vi "MeasureMaxPStab_v2.vi"(7 "Scan Settings JV":T1={"Light intensity (Suns)"=1.0, "Pre-bias time (s)"=0.0, "Maximum voltage (V)"=0.0, "Minimum voltage (V)"=-1.4, "Range Options"=4, "1st scan FB to SC?"=TRUE, "Step Size (V)"=0.01, "Source Delay (s)"=0.01, "Inverted device"=FALSE, "Measure stabilized power output"=TRUE, "Stabilzation time (s)"=40.0, "Use Vmp from JV scan"=TRUE, "Stabization voltage (V)"=0.8, "Only stabilize best pixels"=TRUE, "Number of pixels to stabilize \nper substrate"=0, "Stabilization time step (s)"=1.0, "Use max power tracking"=FALSE, "Pre-bias voltage (V)"=-1.4, "No. of data point averages"=1.0, "No. of J-V averages"=1.0, "Integration time (ms)"=200.0} {"Number of pixels to stabilize \nper substrate" items=["1", "2", "3", "4", "5", "6", "7", "8"]; "Range Options" items=["Auto Range", "100 uA", "1 mA", "10 mA", "100 mA", "1A"]}, 9 "Voltage List":dbl[](array[numeric])) -> (0 "error out":errorcluster, 1 "Data Array":dbl[][](array[numeric]), 3 "VISA resource name out":refnum<visa-resource-name>)   [LabVIEW 2011]
uses:
  Typedefs/Scan settings.ctl
  <instrlib>/Keithley 24XX/Public/Data/Read (Multiple Points).vi
  <instrlib>/Keithley 24XX/Keithley 24XX.lvlib
panel:
  in  "Manual Range (1.0)":dbl=1.0
  in  "Source Mode  (0: Voltage)":u16(ring) items=["Voltage", "Current"]
  in  "VISA resource name":refnum<visa-resource-name>="GPIB0::24::INSTR"
  in  "Number of Points":u32=5
  in  "Compliance  Level":dbl=0.1
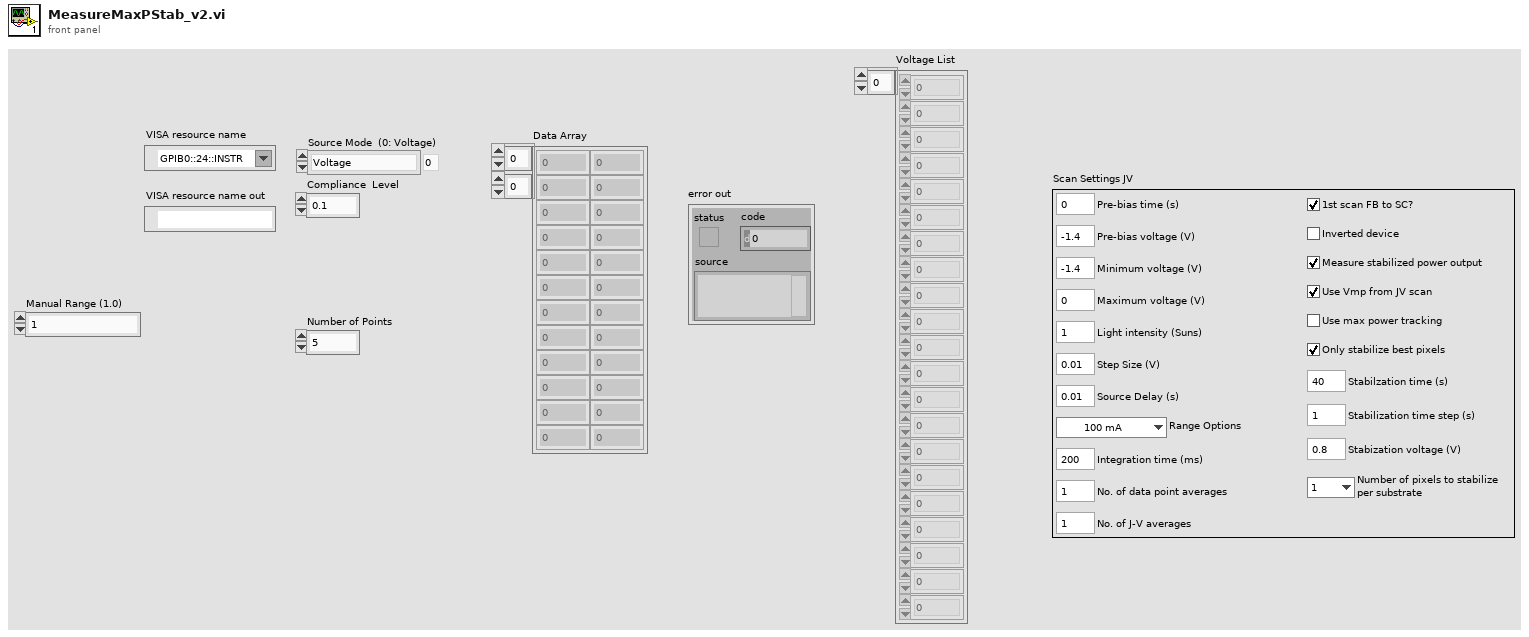
[diagram p1: front panel]
types:
  T1 = typedef "Scan settings.ctl" = cluster{"Light intensity (Suns)":dbl, "Pre-bias time (s)":dbl, "Maximum voltage (V)":dbl, "Minimum voltage (V)":dbl, "Range Options":u16, "1st scan FB to SC?":bool, "Step Size (V)":dbl, "Source Delay (s)":dbl, "Inverted device":bool, "Measure stabilized power output":bool, "Stabilzation time (s)":dbl, "Use Vmp from JV scan":bool, "Stabization voltage (V)":dbl, "Only stabilize best pixels":bool, "Number of pixels to stabilize \nper substrate":u16, "Stabilization time step (s)":dbl, "Use max power tracking":bool, "Pre-bias voltage (V)":dbl, "No. of data point averages":dbl, "No. of J-V averages":dbl, "Integration time (ms)":dbl}
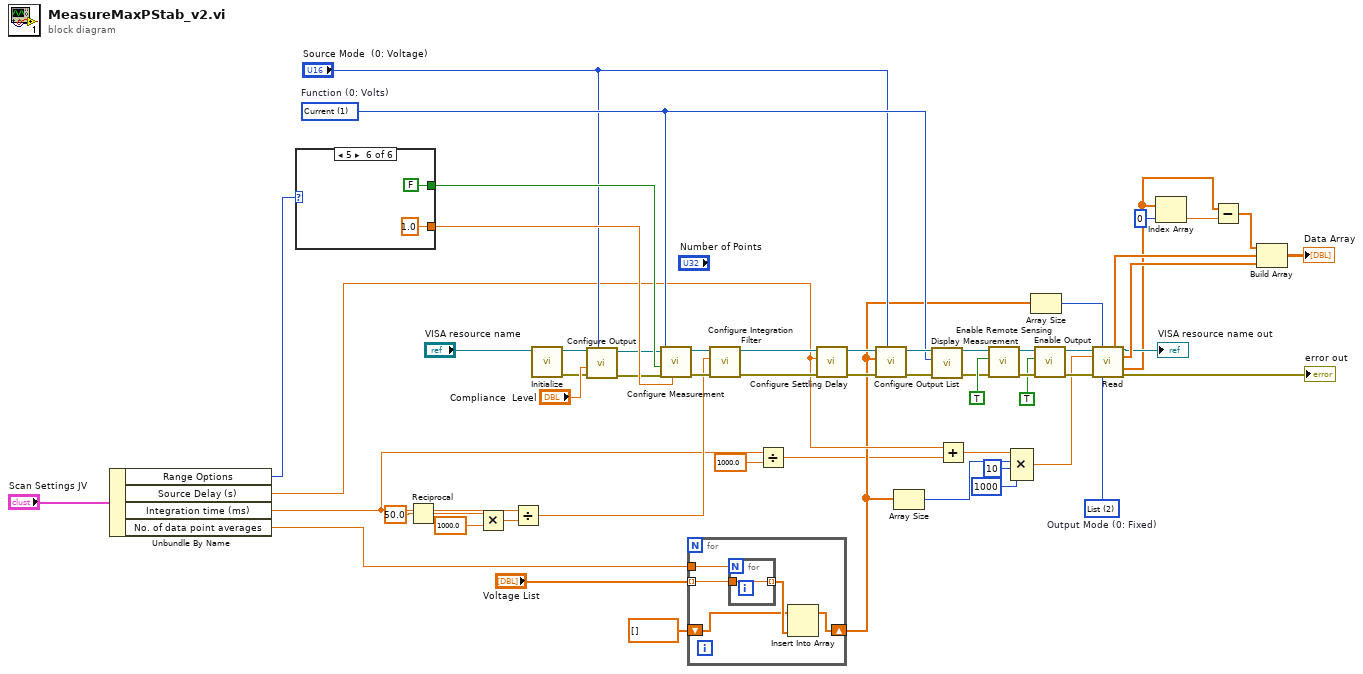
[diagram p0: block diagram]
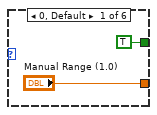
[diagram p2: hidden frame]
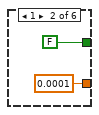
[diagram p3: hidden frame]
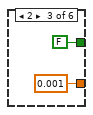
[diagram p4: hidden frame]
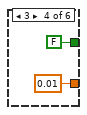
[diagram p5: hidden frame]
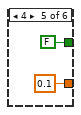
[diagram p6: hidden frame]
diagram:
  w38 = u16 1 items=["Volts", "Current", "Resistance"]  # Function (0: Volts)
  w54 = u16 2 items=["Fixed", "Sweep", "List"]  # Output Mode (0: Fixed)
  n1 = Unbundle By Name("Scan Settings JV") -> ("Range Options"=w24:u16, "Source Delay (s)"=w10:dbl, "Integration time (ms)"=w2:dbl, "No. of data point averages"=w11:dbl)
  n2 = case shown="5" w24 {
    tunnel: ["Manual Range (1.0)" 0.0001 ("Manual Range (1.0)") 0.001 ("Manual Range (1.0)") 0.01 ("Manual Range (1.0)") 0.1 ("Manual Range (1.0)") 1.0 ("Manual Range (1.0)")] -> w25
    tunnel: [TRUE FALSE FALSE FALSE FALSE FALSE] -> w26
    frame 0, Default {
    }
    frame 1 {
    }
    frame 2 {
    }
    frame 3 {
    }
    frame 4 {
    }
    frame 5 {
    }
  }
  n3 = Reciprocal(x=50.0) -> (1/x=w14:dbl)
  n4 = Multiply(x=w14, y=1000.0) -> (x*y=w13:dbl)
  n5 = Divide(x=w2, y=w13) -> (x/y=w12:dbl)
  n6 = call <instrlib>:"Initialize.vi"("VISA resource name"="VISA resource name") -> ("error out"=w21:errorcluster, "VISA resource name out"=w23:refnum<visa-resource-name>)  [unwired: 9 in]
  n7 = call <instrlib>:"Configure Output.vi"("Source Mode  (0: Voltage)"="Source Mode  (0: Voltage)", "error in (no error)"=w21, "Compliance  Level (0.1)"="Compliance  Level", "VISA resource name"=w23) -> ("error out"=w20:errorcluster, "VISA resource name out"=w22:refnum<visa-resource-name>)  [unwired: 6 in]
  n8 = call <instrlib>:"Configure Measurement.vi"("Manual Range (1.0)"=w25, "error in (no error)"=w20, "Enable Auto Range (T:Enable)"=w26, "Function (0: Volts)"=w38, "VISA resource name"=w22) -> ("error out"=w43:errorcluster, "VISA resource name out"=w44:refnum<visa-resource-name>)  [unwired: 5 in]
  n9 = for {
    tunnel: "Voltage List" -> [w74] mode=indexing
    shift-right: [w73] -> w8
    shift-left: dbl[] [] -> [w71]
    tunnel: w11 -> [w70]
    n10 = for {
      N: w70 -> [_]
      tunnel: w74 -> [w75]
      tunnel: [w75] -> w72 mode=indexing
    }
    n11 = Insert Into Array(array=w71, new element=w72) -> (w73:dbl[])  [unwired: 1 in]
  }
  n12 = call <instrlib>:"Configure Integration Filter.vi"("error in (no error)"=w43, "Measurement Speed (1 PLC)"=w12, "VISA resource name"=w44) -> ("error out"=w17:errorcluster, "VISA resource name out"=w18:refnum<visa-resource-name>)  [unwired: 7 in]
  n13 = Divide(x=w2, y=1000.0) -> (x/y=w3:dbl)
  n14 = call <instrlib>:"Configure Settling Delay.vi"("error in (no error)"=w17, "Manual Settling Delay (0 sec)"=w10, "VISA resource name"=w18) -> ("error out"=w35:errorcluster, "VISA resource name out"=w36:refnum<visa-resource-name>)  [unwired: 7 in]
  n15 = call <instrlib>:"Configure Output List.vi"("Source Mode  (0: Voltage)"="Source Mode  (0: Voltage)", "error in (no error)"=w35, "Output List"=w8, "VISA resource name"=w36) -> ("error out"=w41:errorcluster, "VISA resource name out"=w42:refnum<visa-resource-name>)  [unwired: 6 in]
  n16 = Array Size(array=w8) -> (size(s)=w7:i32)
  n17 = call <instrlib>:"Display Measurement.vi"("error in (no error)"=w41, "Displayed Measurement (0: Voltage)"=w38, "VISA resource name"=w42) -> ("error out"=w39:errorcluster, "VISA resource name out"=w40:refnum<visa-resource-name>)  [unwired: 7 in]
  n18 = Add(x=w10, y=w3) -> (x+y=w9:dbl)
  n19 = call <instrlib>:"Enable Remote Sensing.vi"("error in (no error)"=w39, "Enable Remote Sensing (T: Enable)"=TRUE ("Enable Output (T: Enable)"), "VISA resource name"=w40) -> ("error out"=w48:errorcluster, "VISA resource name out"=w49:refnum<visa-resource-name>)  [unwired: 7 in]
  n20 = Compound Arithmetic op=MULTIPLY(w9, w7, 10 ("value"), 1000 ("value")) -> (w5:dbl)
  n21 = Array Size(array=w8) -> (size(s)=w34:i32)
  n22 = call <instrlib>:"Enable Output.vi"("error in (no error)"=w48, "Enable Output (T: Enable)"=TRUE, "VISA resource name"=w49) -> ("error out"=w53:errorcluster, "VISA resource name out"=w52:refnum<visa-resource-name>)  [unwired: 7 in]
  n23 = call-poly <instrlib>:"Read.vi"("VISA resource name"=w52, "Sample Count (1)"=w34, "Timeout (10000 ms)"=w5, "error in (no error)"=w53, "Output Mode (0: Fixed)"=w54) -> ("Voltage"=w56:sgl[], "VISA resource name out"=→"VISA resource name out":refnum<visa-resource-name>, "Current"=w55:sgl[], "Timestamp"=w31:sgl[], "error out"=→"error out":errorcluster)  [unwired: 4 in, 2 out]
  n24 = Index Array(array=w31, index=0) -> (element=w32:sgl)
  n25 = Subtract(x=w31, y=w32) -> (x-y=w30:sgl[])
  n26 = Build Array(w30, w56, w55) -> (→"Data Array":sgl[][])
